vi "PH_ImageOperator.panel.vi"(0 "object ref":refnum<vi>, 5 "error in (no error)":errorcluster) -> (19 "error out":errorcluster)   [LabVIEW 2014, in "PH_ImageOperator.lvlib"]
doc: "The voltage measured by a device on high potential is represented by a frequency given out by a Beckhoff Klemme. This VI transforms it back into a voltage which wich is written to a memory tag. This value is indicated. In case of no connection (not mounted or bad tag value) or internal problems \"99999\" apears.\n\n\"Exit\" closes the GUI while \"Delete Instance\" additionally destroys the Instance.\n\n\n\nLicense Agreement for this software:\n\nCopyright (C)\nGesellschaft für Schwerionenforschung, GSI\nPlanckstr. 1\n64291 Darmstadt\nGermany\n\nContact: D.Beck@gsi.de \n\nThis program is free software; you can redistribute it and/or modify it under the terms of the GNU General Public License as published by the Free Software Foundation; either version 2 of the license, or (at your option) any later version.\n\nThis program is distributed in the hope that it will be useful, but WITHOUT ANYW ARRANTY; without even the implied warranty of MERCHANTABILITY or FITNESS FOR A PARTICULAR PURPOSE. See the GNU General License for more details (http://www.gnu.org).\n\nGesellschaft für Schwerionenforschung, GSI\nPlanckstr. 1, 64291 Darmstadt, Germany\nFor all questions and ideas contact: M.Richter@gsi.de, H.Brand@gsi.de or D.Beck@gsi.de.\nLast update: 18-DEC-2002"
uses:
  PH_ImageOperator.lvlib
  PH_ImageCalibrator/PH_ImageCalibrator.Calibration Data.ctl
  PH_Basics/PH_Img_BaseClass/PH_Img_BaseClass.Palette.ctl
  PH_Basics/PH_Img_BaseClass/PH_Img_BaseClass.GUI Refs.ctl
  CS_Core/CSObj/CSObj.lvlib
  CS_Core/CSSystem/CSSystemLib/CSSystemLib.lvlib
  PH_Basics/PH_Common/PH_Common.lvlib
  PH_Basics/PH_Img_BaseClass/PH_Img_BaseClass.lvlib
  PH_Basics/PH_Class/PH_Class.lvlib
  PH_Basics/PH_PSDBWriter/PH_PSDBWriter.lvlib
  PH_ImageCalibrator/PH_ImageCalibrator.lvlib
panel:
  out "PSDB Status":u32(colorbox)=6618880 caption="PSDB"
  in  "M":dbl
  in  "f 2":dbl caption="mm"
  out "Calibration status":u32(colorbox)=16860 caption="Calibration"
  out "Timeout":u32(colorbox)=16860
  in  "Tab Control":T1(tab)
  in  "Filter":bool
  in  "Damage Threshold":dbl=3.0 caption="J/cm²"
  in  "FF: Threshold":dbl=0.13 caption="Threshold"
  out "max. allowed Energy":dbl caption="J"
  out "Fillfactor":dbl
  out "Fill Factor calculated":u32(colorbox)=16860 caption="Fill Factor"
  in  "calc Fill Factor":bool caption="Fill Factor"
  out "Min 1 %":dbl caption="Pix"
  out "Maj 1 %":dbl caption="Pix"
  in  "Traces: No Offset":bool caption="No Offset"
  out "Traces calculated":u32(colorbox)=16860 caption="Trace"
  in  "Traces: Fit Gauss":bool caption="Fit Gauss"
  out "Min Fit Order":i32
  out "Maj Fit Order":i32
  out "Min FWHM":dbl caption="Pix"
  out "Maj FWHM":dbl caption="Pix"
  in  "Traces":bool
  in  "Timeout Set":i32 caption="ms"
  in  "Global On":bool caption="On"
  out "BI subtracted":u32(colorbox)=16860
  out "D":dbl caption="mm"
  out "q":dbl caption="mrad"
  in  "Center":bool
  in  "exp - Y":i32 caption="Pix"
  in  "Tolerance":dbl caption="mrad"
  in  "exp - X":i32 caption="Pix"
  out "Position calculated":u32(colorbox)=16860 caption="Position"
  in  "Type":bool
  in  "Position":bool
  out "Dummy Type":bool caption="NF       FF"
  in  "BA: Method":bool caption="Method"
  in  "BA: Factor for ROI":i32=3 caption="Factor"
  in  "BA: Steps":i32=3 caption="Steps"
  out "CoG - Y":dbl caption="Pix"
  out "CoG - X":dbl caption="Pix"
  out "e":dbl caption="PixSum"
  out "f":dbl caption="°"
  out "Min Diam":dbl caption="Pix"
  out "Maj Diam":dbl caption="Pix"
  out "Beam analysed":u32(colorbox)=16860 caption="Beam Analysis"
  in  "calc Beam Analysis":bool caption="Analysis"
  out "Dummy Method":bool caption="OA     ROI"
  out "Energy":dbl caption="PiS" format="%#_8g"
  out "Energy calculated":u32(colorbox)=16860 caption="Energy"
  in  "Tolerance":dbl caption="%"
  in  "expected":dbl caption="mJ"
  in  "calc Energy":bool caption="Energy"
  out "Minor Trace":cluster{"Index":sgl[], dbl[]}[](graph)
  out "Major Trace":cluster{"Index":sgl[], dbl[]}[](graph)
  in  "Palette":T2 items=["Grey", "Binary", "Gradient", "Rainbow", "Temperature"]
  out "GUI Image":T3(plugin-control)
  out "GUI FF Image":T3(plugin-control)
  in  "read calibration data":bool
  out "Calibration data":T4
  in  "Exit":bool
  in  "Delete":bool
  # "PCS"
  # "3.40"
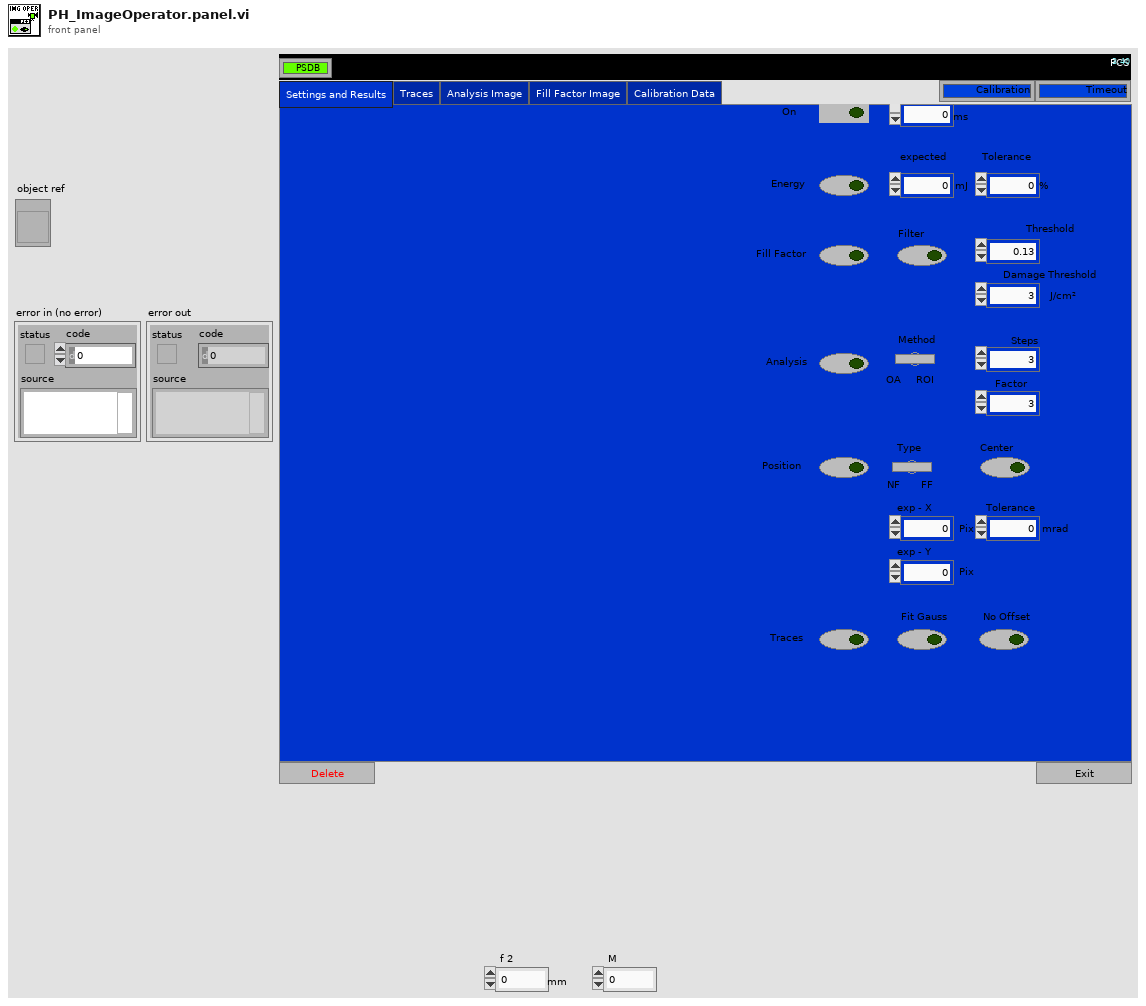
[diagram p1: front panel]
types:
  T1 = enum32{"Settings and Results", "Traces", "Analysis Image", "Fill Factor Image", "Calibration Data"}
  T2 = typedef "PH_Img_BaseClass.lvlib/PH_Img_BaseClass.Palette.ctl" = i32
  T3 = typedef "IMAQ Image.ctl" = refnum<image>
  T4 = typedef "PH_ImageCalibrator.lvlib/PH_ImageCalibrator.Calibration Data.ctl" = cluster{"Date":string, "Time":string, "Cam Settings":cluster{"Cam ID":string, "Gain":dbl, "Brightness":dbl, "Shutter":dbl, "Cam Error":bool, "Mode":i32}, "Background Image":cluster{"Image":dbl[][], "Image Error":bool}, "Linear Calibration":cluster{"Calibration Factor":dbl, "not mm or mrad":bool}, "Energy Calibration":cluster{"Calibration Factor":dbl, "no mJ":bool}}
  T5 = typedef "PH_Img_BaseClass.lvlib/PH_Img_BaseClass.GUI Refs.ctl" = cluster{"Timeout":refnum<vi>, "Image":refnum<vi>, "Palette":refnum<vi>, "Timeout Set":refnum<vi>}
  T6 = typedef "PH_ImageOperator.lvlib/PH_ImageOperator.i attribute.ctl" = cluster{"GUI Refs":cluster{"Delete":refnum<vi>, "Calibration status":refnum<vi>, "BI subtracted":refnum<vi>, "calc Energy":refnum<vi>, "Energy: expected value":refnum<vi>, "Energy: Tolerance":refnum<vi>, "Energy calculated":refnum<vi>, "Energy":refnum<vi>, "calc Beam Anal":refnum<vi>, "Maj Diam 1/esquare":refnum<vi>, "Min Diam 1/esquare":refnum<vi>, "Azi Angle":refnum<vi>, "Min/Maj Diam esquare":refnum<vi>, "Beam analysed":refnum<vi>, "CoG - x":refnum<vi>, "CoG - y":refnum<vi>, "BA: Method":refnum<vi>, "BA: Steps":refnum<vi>, "BA: Factor":refnum<vi>, "calc Traces":refnum<vi>, "Traces: Fit Gauss":refnum<vi>, "Traces calculated":refnum<vi>, "Maj FWHM":refnum<vi>, "Min FWHM":refnum<vi>, "Major Trace":refnum<vi>, "Minor Trace":refnum<vi>, "Maj Fit Order":refnum<vi>, "Min Fit Order":refnum<vi>, "Position calculated":refnum<vi>, "Position":refnum<vi>, "Type":refnum<vi>, "Center":refnum<vi>, "exp - X":refnum<vi>, "exp - Y":refnum<vi>, "Tolerance":refnum<vi>, "f":refnum<vi>, "M":refnum<vi>, "D":refnum<vi>, "q":refnum<vi>, "Dummy Method":refnum<vi>, "Dummy Type":refnum<vi>, "Global On":refnum<vi>, "Traces: No offset":refnum<vi>, "Maj 99%":refnum<vi>, "Min 99%":refnum<vi>, "GUI FF Image":refnum<vi>, "calc Fill Factor":refnum<vi>, "FF calculated":refnum<vi>, "Fill Factor: Filter?":refnum<vi>, "FF: Damage Threshold":refnum<vi>, "FF: Threshold":refnum<vi>, "FF: max allow. Energy":refnum<vi>, "FF: Fillfactor":refnum<vi>, "Calibration data":refnum<vi>}, "List of GUIs":string[], "Calibration":cluster{"Status":T7, "Calibration data":T4, "Calibration Data File":path}, "Final Image":cluster{"BI Subtraction Failure":bool}, "Energy":cluster{"on":bool, "expected value [mJ]":dbl, "Tolerance [%]":dbl, "State":T7, "Energy [mJ]":dbl, "Unit":string, "calculated @":timestamp}, "Beam Analysis":cluster{"on":bool, "Data":T8, "Method":bool, "Steps":i32, "Factor":i32, "ROI":cluster{"Left":i32, "Top":i32, "Right":i32, "Bottom":i32}, "analysed @":timestamp}, "Trace Analysis":cluster{"on":bool, "Fit on":bool, "Maj FWHM":dbl, "Min FWHM":dbl, "Maj Fit Order":i32, "Min Fit Order":i32, "No Offset":bool, "Maj 99%":dbl, "Min 99%":dbl, "Traces":cluster{"XScaleName":string, "Y Scale Minimum":sgl, "Y Scale Maximum":sgl, "X Scale Minimum":sgl, "X Scale Maximum":sgl, "Traces":cluster{"Index":sgl[], "Trace":dbl[]}[]}[], "analysed @":timestamp}, "Position Analysis":cluster{"on":bool, "exp - X":i32, "exp - Y":i32, "focal length [mm]":dbl, "Magnification":dbl, "Delta":dbl, "Theta":dbl, "Tolerance":dbl, "Type":bool, "analysed @":timestamp}, "Fill Factor":cluster{"on":bool, "Filter on?":bool, "Threshold":dbl, "Damage Threshold [J/cm²]":dbl, "Fillfactor":dbl, "Max. allowed Energy [J]":dbl, "calculated @":timestamp}, "Statistician Service ID":i32, "Images":cluster{"Background":T3, "OP":T3, "GUI":T3, "BA: ROI":T3, "Trace: Turn":T3, "FF: Main":T3, "FF: Help":T3, "PSDB: BG":T3, "PSDB: OP":T3, "PSDB: FF":T3}}
  T7 = typedef "PH_StatusHandler.lvlib/PH_StatusHandler.Status.ctl" = i16
  T8 = typedef "PH_ImageOperator.lvlib/PH_ImageOperator.Beam Analysis Data.ctl" = cluster{"CoG-x":sgl, "CoG-y":sgl, "Maj Dim":dbl, "Min Dim":dbl, "Ellipticity":dbl, "Azimuth Angle [rad]":dbl, "Azi Angle rel to Maj?":bool}
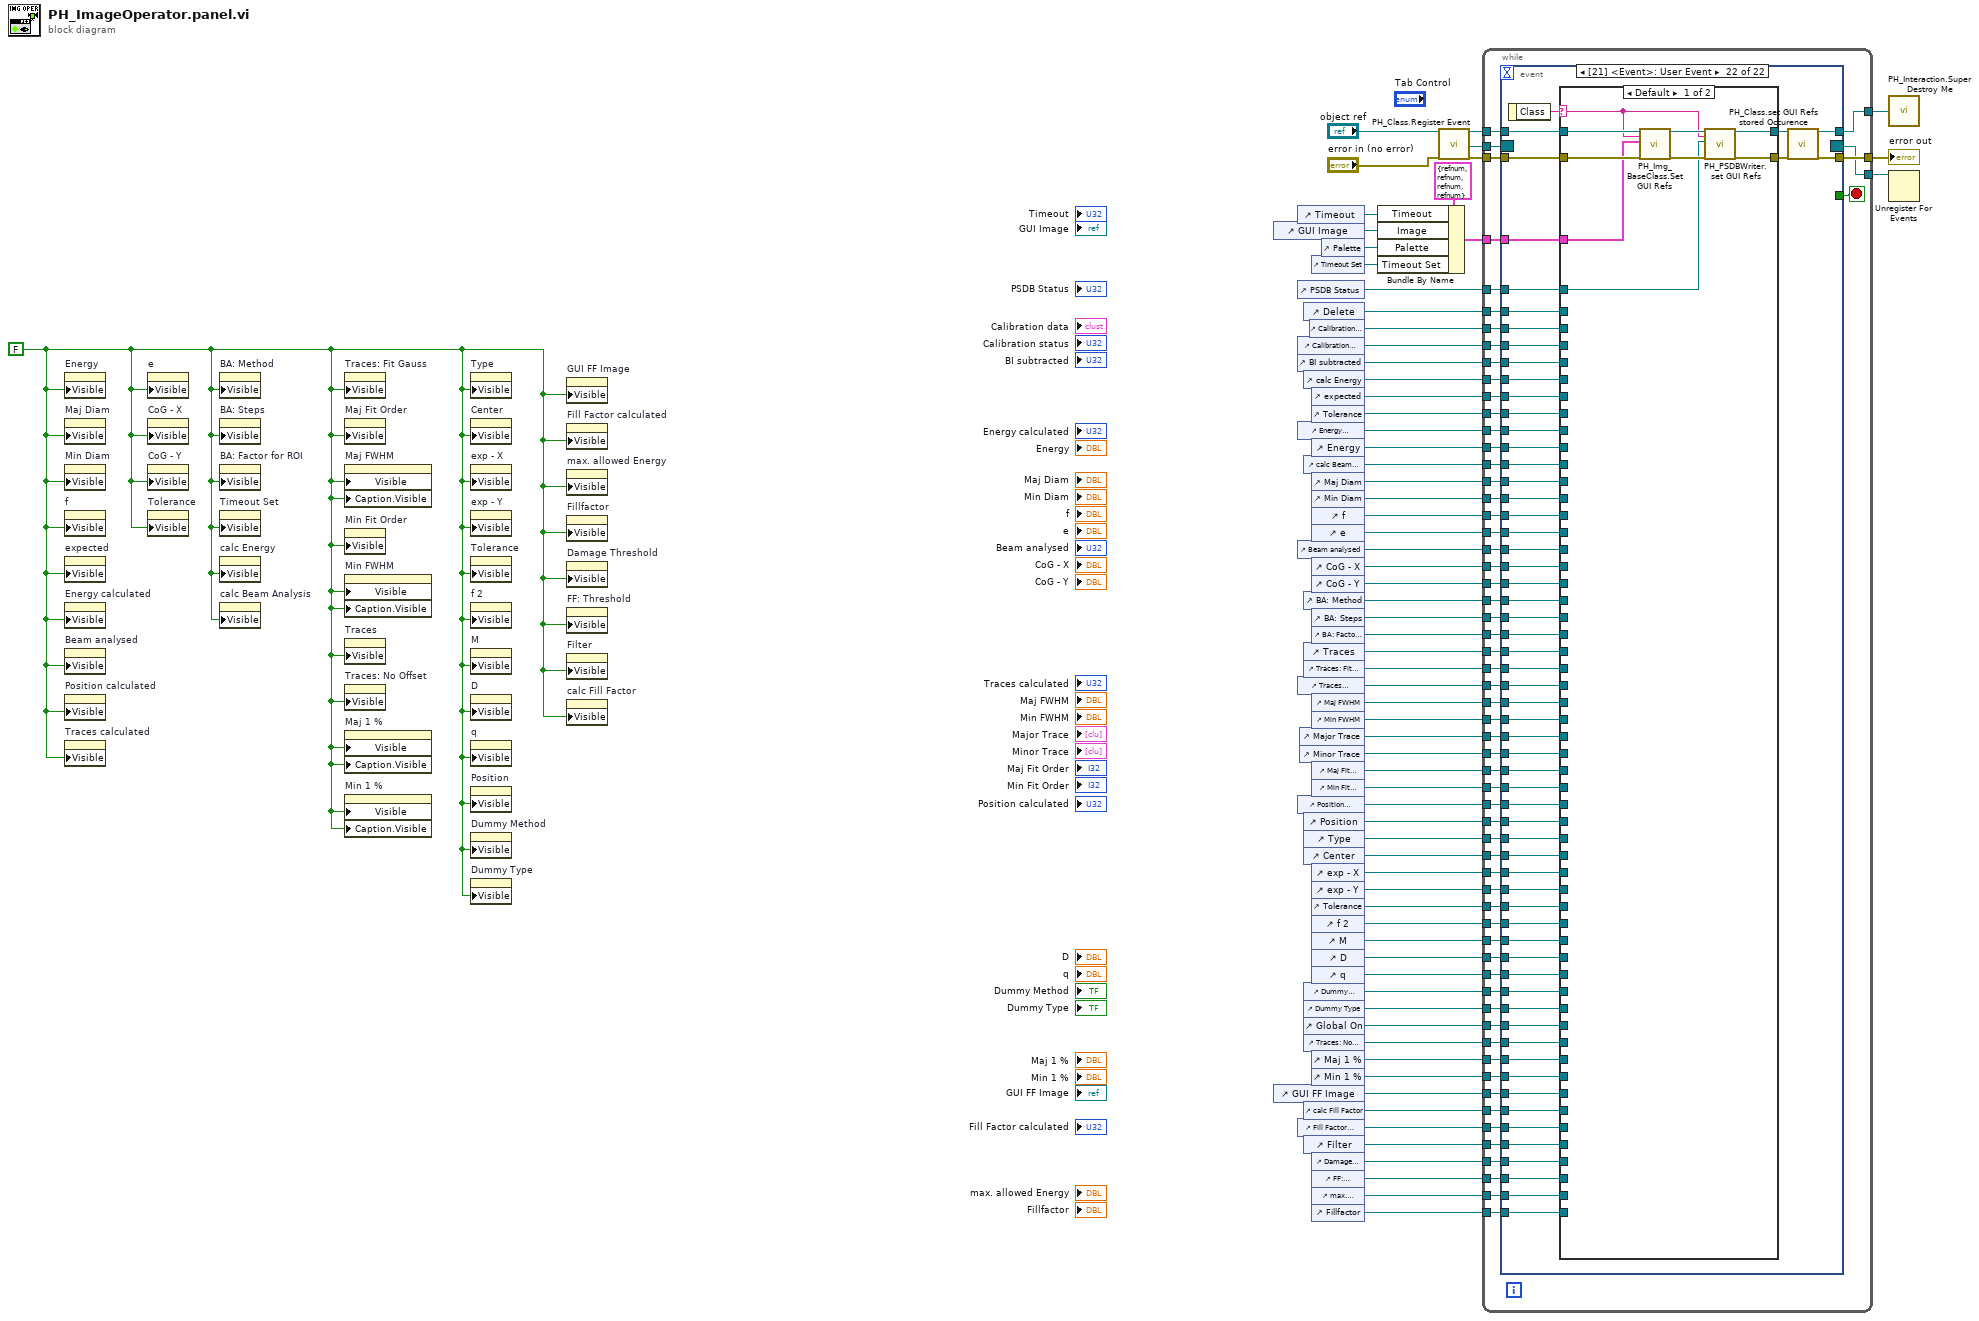
[diagram p0: block diagram]
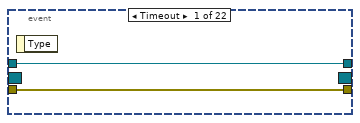
[diagram p2: hidden frame]
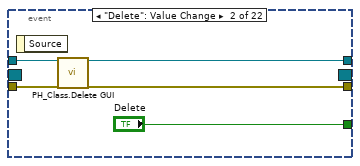
[diagram p3: hidden frame]
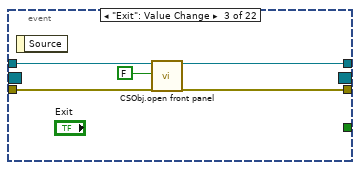
[diagram p4: hidden frame]
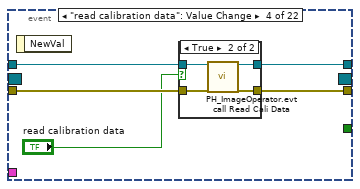
[diagram p5: hidden frame]
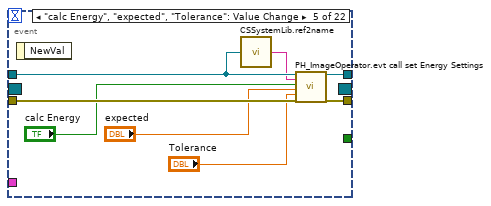
[diagram p7: hidden frame]
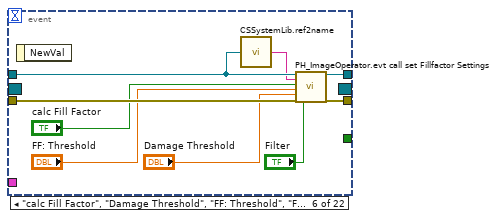
[diagram p8: hidden frame]
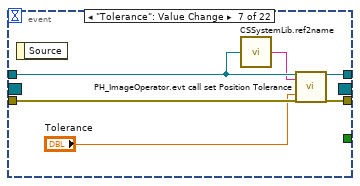
[diagram p9: hidden frame]
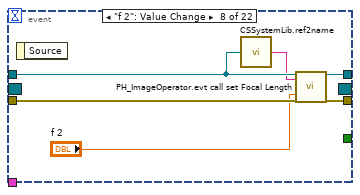
[diagram p10: hidden frame]
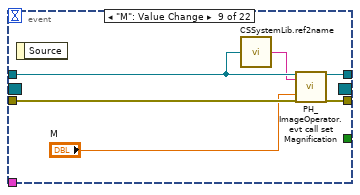
[diagram p11: hidden frame]
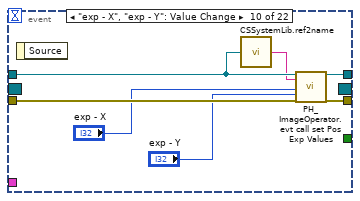
[diagram p12: hidden frame]
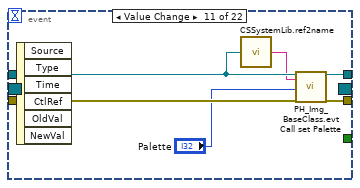
[diagram p13: hidden frame]
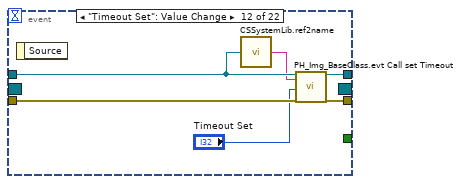
[diagram p14: hidden frame]
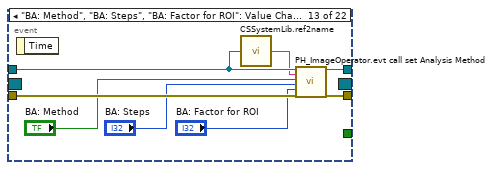
[diagram p15: hidden frame]
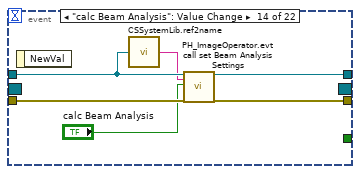
[diagram p16: hidden frame]
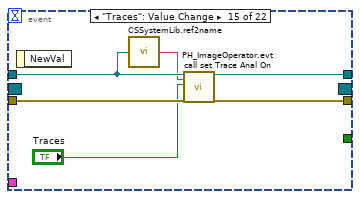
[diagram p17: hidden frame]
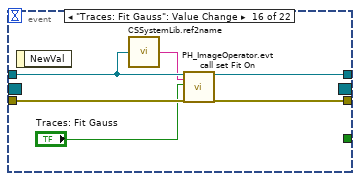
[diagram p18: hidden frame]
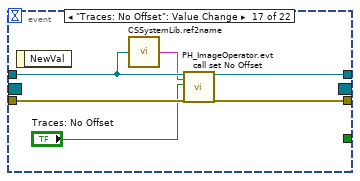
[diagram p19: hidden frame]
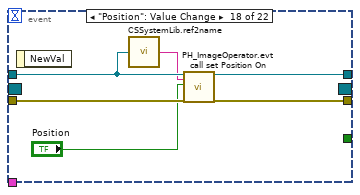
[diagram p20: hidden frame]
diagram:
  w68 = FALSE
  n1 = property on="Energy" class="DigNum (strict)"("Visible"=w68) -> ()  [unwired: 2 in, 2 out]
  n2 = property on="Maj Diam" class="DigNum (strict)"("Visible"=w68) -> ()  [unwired: 2 in, 2 out]
  n3 = property on="Min Diam" class="DigNum (strict)"("Visible"=w68) -> ()  [unwired: 2 in, 2 out]
  n4 = property on="f" class="DigNum (strict)"("Visible"=w68) -> ()  [unwired: 2 in, 2 out]
  n5 = property on="expected" class="DigNum (strict)"("Visible"=w68) -> ()  [unwired: 2 in, 2 out]
  n6 = property on="Energy calculated" class="ColBox"("Visible"=w68) -> ()  [unwired: 2 in, 2 out]
  n7 = property on="Beam analysed" class="ColBox"("Visible"=w68) -> ()  [unwired: 2 in, 2 out]
  n8 = property on="Position calculated" class="ColBox"("Visible"=w68) -> ()  [unwired: 2 in, 2 out]
  n9 = property on="Traces calculated" class="ColBox"("Visible"=w68) -> ()  [unwired: 2 in, 2 out]
  n10 = property on="e" class="DigNum (strict)"("Visible"=w68) -> ()  [unwired: 2 in, 2 out]
  n11 = property on="CoG - X" class="DigNum (strict)"("Visible"=w68) -> ()  [unwired: 2 in, 2 out]
  n12 = property on="CoG - Y" class="DigNum (strict)"("Visible"=w68) -> ()  [unwired: 2 in, 2 out]
  n13 = property on="Tolerance" class="DigNum (strict)"("Visible"=w68) -> ()  [unwired: 2 in, 2 out]
  n14 = property on="BA: Method" class="Bool (strict)"("Visible"=w68) -> ()  [unwired: 2 in, 2 out]
  n15 = property on="BA: Steps" class="DigNum (strict)"("Visible"=w68) -> ()  [unwired: 2 in, 2 out]
  n16 = property on="BA: Factor for ROI" class="DigNum (strict)"("Visible"=w68) -> ()  [unwired: 2 in, 2 out]
  n17 = property on="Timeout Set" class="DigNum (strict)"("Visible"=w68) -> ()  [unwired: 2 in, 2 out]
  n18 = property on="calc Energy" class="Bool (strict)"("Visible"=w68) -> ()  [unwired: 2 in, 2 out]
  n19 = property on="calc Beam Analysis" class="Bool (strict)"("Visible"=w68) -> ()  [unwired: 2 in, 2 out]
  n20 = property on="Traces: Fit Gauss" class="Bool (strict)"("Visible"=w68) -> ()  [unwired: 2 in, 2 out]
  n21 = property on="Maj Fit Order" class="DigNum (strict)"("Visible"=w68) -> ()  [unwired: 2 in, 2 out]
  n22 = property on="Maj FWHM" class="DigNum (strict)"("Visible"=w68, "Caption.Visible"=w68) -> ()  [unwired: 2 in, 2 out]
  n23 = property on="Min Fit Order" class="DigNum (strict)"("Visible"=w68) -> ()  [unwired: 2 in, 2 out]
  n24 = property on="Min FWHM" class="DigNum (strict)"("Visible"=w68, "Caption.Visible"=w68) -> ()  [unwired: 2 in, 2 out]
  n25 = property on="Traces" class="Bool (strict)"("Visible"=w68) -> ()  [unwired: 2 in, 2 out]
  n26 = property on="Traces: No Offset" class="Bool (strict)"("Visible"=w68) -> ()  [unwired: 2 in, 2 out]
  n27 = property on="Maj 1 %" class="DigNum (strict)"("Visible"=w68, "Caption.Visible"=w68) -> ()  [unwired: 2 in, 2 out]
  n28 = property on="Min 1 %" class="DigNum (strict)"("Visible"=w68, "Caption.Visible"=w68) -> ()  [unwired: 2 in, 2 out]
  n29 = property on="Type" class="Bool (strict)"("Visible"=w68) -> ()  [unwired: 2 in, 2 out]
  n30 = property on="Center" class="Bool (strict)"("Visible"=w68) -> ()  [unwired: 2 in, 2 out]
  n31 = property on="exp - X" class="DigNum (strict)"("Visible"=w68) -> ()  [unwired: 2 in, 2 out]
  n32 = property on="exp - Y" class="DigNum (strict)"("Visible"=w68) -> ()  [unwired: 2 in, 2 out]
  n33 = property on="Tolerance" class="DigNum (strict)"("Visible"=w68) -> ()  [unwired: 2 in, 2 out]
  n34 = property on="f 2" class="DigNum (strict)"("Visible"=w68) -> ()  [unwired: 2 in, 2 out]
  n35 = property on="M" class="DigNum (strict)"("Visible"=w68) -> ()  [unwired: 2 in, 2 out]
  n36 = property on="D" class="DigNum (strict)"("Visible"=w68) -> ()  [unwired: 2 in, 2 out]
  n37 = property on="q" class="DigNum (strict)"("Visible"=w68) -> ()  [unwired: 2 in, 2 out]
  n38 = property on="Position" class="Bool (strict)"("Visible"=w68) -> ()  [unwired: 2 in, 2 out]
  n39 = property on="Dummy Method" class="Bool (strict)"("Visible"=w68) -> ()  [unwired: 2 in, 2 out]
  n40 = property on="Dummy Type" class="Bool (strict)"("Visible"=w68) -> ()  [unwired: 2 in, 2 out]
  n41 = property on="GUI FF Image" class="ImageControl"("Visible"=w68) -> ()  [unwired: 2 in, 2 out]
  n42 = property on="Fill Factor calculated" class="ColBox"("Visible"=w68) -> ()  [unwired: 2 in, 2 out]
  n43 = property on="max. allowed Energy" class="DigNum (strict)"("Visible"=w68) -> ()  [unwired: 2 in, 2 out]
  n44 = property on="Fillfactor" class="DigNum (strict)"("Visible"=w68) -> ()  [unwired: 2 in, 2 out]
  n45 = property on="Damage Threshold" class="DigNum (strict)"("Visible"=w68) -> ()  [unwired: 2 in, 2 out]
  n46 = property on="FF: Threshold" class="DigNum (strict)"("Visible"=w68) -> ()  [unwired: 2 in, 2 out]
  n47 = property on="Filter" class="Bool (strict)"("Visible"=w68) -> ()  [unwired: 2 in, 2 out]
  n48 = property on="calc Fill Factor" class="Bool (strict)"("Visible"=w68) -> ()  [unwired: 2 in, 2 out]
  n49 = control-ref of="GUI Image"() -> (w65:refnum<vi>)
  n50 = control-ref of="GUI FF Image"() -> (w8:refnum<vi>)
  n51 = control-ref of="Timeout"() -> (w66:refnum<vi>)
  n52 = control-ref of="PSDB Status"() -> (w57:refnum<vi>)
  n53 = control-ref of="Calibration status"() -> (w52:refnum<vi>)
  n54 = control-ref of="BI subtracted"() -> (w51:refnum<vi>)
  n55 = control-ref of="Energy calculated"() -> (w47:refnum<vi>)
  n56 = control-ref of="Beam analysed"() -> (w40:refnum<vi>)
  n57 = control-ref of="Traces calculated"() -> (w32:refnum<vi>)
  n58 = control-ref of="Position calculated"() -> (w25:refnum<vi>)
  n59 = control-ref of="Fill Factor calculated"() -> (w6:refnum<vi>)
  n60 = control-ref of="Major Trace"() -> (w29:refnum<vi>)
  n61 = control-ref of="Minor Trace"() -> (w28:refnum<vi>)
  n62 = control-ref of="Delete"() -> (w56:refnum<vi>)
  n63 = control-ref of="calc Energy"() -> (w50:refnum<vi>)
  n64 = control-ref of="calc Beam Analysis"() -> (w45:refnum<vi>)
  n65 = control-ref of="BA: Method"() -> (w37:refnum<vi>)
  n66 = control-ref of="Traces"() -> (w34:refnum<vi>)
  n67 = control-ref of="Traces: Fit Gauss"() -> (w33:refnum<vi>)
  n68 = control-ref of="Position"() -> (w24:refnum<vi>)
  n69 = control-ref of="Type"() -> (w23:refnum<vi>)
  n70 = control-ref of="Center"() -> (w22:refnum<vi>)
  n71 = control-ref of="Dummy Method"() -> (w14:refnum<vi>)
  n72 = control-ref of="Dummy Type"() -> (w13:refnum<vi>)
  n73 = control-ref of="Global On"() -> (w12:refnum<vi>)
  n74 = control-ref of="Traces: No Offset"() -> (w11:refnum<vi>)
  n75 = control-ref of="calc Fill Factor"() -> (w7:refnum<vi>)
  n76 = control-ref of="Filter"() -> (w5:refnum<vi>)
  n77 = control-ref of="Calibration data"() -> (w53:refnum<vi>)
  n78 = control-ref of="Timeout Set"() -> (w63:refnum<vi>)
  n79 = control-ref of="expected"() -> (w49:refnum<vi>)
  n80 = control-ref of="Tolerance"() -> (w48:refnum<vi>)
  n81 = control-ref of="Energy"() -> (w46:refnum<vi>)
  n82 = control-ref of="Maj Diam"() -> (w44:refnum<vi>)
  n83 = control-ref of="Min Diam"() -> (w43:refnum<vi>)
  n84 = control-ref of="f"() -> (w42:refnum<vi>)
  n85 = control-ref of="e"() -> (w41:refnum<vi>)
  n86 = control-ref of="CoG - X"() -> (w39:refnum<vi>)
  n87 = control-ref of="CoG - Y"() -> (w38:refnum<vi>)
  n88 = control-ref of="BA: Steps"() -> (w36:refnum<vi>)
  n89 = control-ref of="BA: Factor for ROI"() -> (w35:refnum<vi>)
  n90 = control-ref of="Maj FWHM"() -> (w31:refnum<vi>)
  n91 = control-ref of="Min FWHM"() -> (w30:refnum<vi>)
  n92 = control-ref of="Maj Fit Order"() -> (w27:refnum<vi>)
  n93 = control-ref of="Min Fit Order"() -> (w26:refnum<vi>)
  n94 = control-ref of="exp - X"() -> (w21:refnum<vi>)
  n95 = control-ref of="exp - Y"() -> (w20:refnum<vi>)
  n96 = control-ref of="Tolerance"() -> (w19:refnum<vi>)
  n97 = control-ref of="f 2"() -> (w18:refnum<vi>)
  n98 = control-ref of="M"() -> (w17:refnum<vi>)
  n99 = control-ref of="D"() -> (w16:refnum<vi>)
  n100 = control-ref of="q"() -> (w15:refnum<vi>)
  n101 = control-ref of="Maj 1 %"() -> (w10:refnum<vi>)
  n102 = control-ref of="Min 1 %"() -> (w9:refnum<vi>)
  n103 = control-ref of="Damage Threshold"() -> (w4:refnum<vi>)
  n104 = control-ref of="FF: Threshold"() -> (w3:refnum<vi>)
  n105 = control-ref of="max. allowed Energy"() -> (w2:refnum<vi>)
  n106 = control-ref of="Fillfactor"() -> (w1:refnum<vi>)
  n107 = control-ref of="Palette"() -> (w64:refnum<vi>)
  n108 = Bundle By Name(cluster=T5 {"Timeout"=refnum, "Image"=refnum, "Palette"=refnum, "Timeout Set"=refnum} ("GUI Refs"), "Timeout"=w66, "Image"=w65, "Palette"=w64, "Timeout Set"=w63) -> (w58:T5)
  n109 = call "PH_Class.Register Event.vi"("i ref in"="object ref", "error in (no error)"="error in (no error)") -> ("i ref out"=w60:refnum<vi>, "Event Registration Refnum"=w59:refnum<event-registration>, "error out"=w61:errorcluster)  [unwired: 15 in]
  n110 = while {
    tunnel: w60 -> [w130]
    tunnel: [w129] -> w70
    tunnel: w61 -> [w132]
    tunnel: [w131] -> w69
    tunnel: [w128] -> w62
    tunnel: w59 -> [w127]
    tunnel: w58 -> [w126]
    tunnel: w57 -> [w125]
    tunnel: w56 -> [w124]
    tunnel: w53 -> [w123]
    tunnel: w52 -> [w122]
    tunnel: w51 -> [w121]
    tunnel: w50 -> [w120]
    tunnel: w49 -> [w119]
    tunnel: w48 -> [w118]
    tunnel: w47 -> [w117]
    tunnel: w46 -> [w116]
    tunnel: w45 -> [w115]
    tunnel: w44 -> [w114]
    tunnel: w43 -> [w113]
    tunnel: w42 -> [w112]
    tunnel: w41 -> [w111]
    tunnel: w40 -> [w110]
    tunnel: w39 -> [w109]
    tunnel: w38 -> [w108]
    tunnel: w37 -> [w107]
    tunnel: w36 -> [w106]
    tunnel: w35 -> [w105]
    tunnel: w34 -> [w104]
    tunnel: w33 -> [w103]
    tunnel: w32 -> [w102]
    tunnel: w31 -> [w101]
    tunnel: w30 -> [w100]
    tunnel: w29 -> [w99]
    tunnel: w28 -> [w98]
    tunnel: w27 -> [w97]
    tunnel: w26 -> [w96]
    tunnel: w25 -> [w95]
    tunnel: w24 -> [w94]
    tunnel: w23 -> [w93]
    tunnel: w22 -> [w92]
    tunnel: w21 -> [w91]
    tunnel: w20 -> [w90]
    tunnel: w19 -> [w89]
    tunnel: w18 -> [w88]
    tunnel: w17 -> [w87]
    tunnel: w16 -> [w86]
    tunnel: w15 -> [w85]
    tunnel: w14 -> [w84]
    tunnel: w13 -> [w83]
    tunnel: w12 -> [w82]
    tunnel: w11 -> [w81]
    tunnel: w10 -> [w80]
    tunnel: w9 -> [w79]
    tunnel: w8 -> [w78]
    tunnel: w7 -> [w77]
    tunnel: w6 -> [w76]
    tunnel: w5 -> [w75]
    tunnel: w4 -> [w74]
    tunnel: w3 -> [w73]
    tunnel: w2 -> [w72]
    tunnel: w1 -> [w71]
    stop <- w133 stop-if-true
    n111 = event shown="[21] <Event>: User Event" {
      selector: w127 -> [_ _ _ _ _ _ _ _ _ _ _ _ _ _ _ _ _ _ _ _ _ _]
      dyn-events: [_ _ _ _ _ _ _ _ _ _ _ _ _ _ _ _ _ _ _ _ _ _] -> w128
      timeout: _ -> [_ _ _ _ _ _ _ _ _ _ _ _ _ _ _ _ _ _ _ _ _ _]
      tunnel: [_ "Delete" _ _ _ _ _ _ _ _ _ _ _ _ _ _ _ _ _ _ _ _] -> w133
      tunnel: w130 -> [w134 w138 w144 w150 w161 w170 w176 w182 w188 w195 w201 w207 w215 w221 w227 w233 w239 w245 w251 w257 w262 w328]
      tunnel: w132 -> [w135 w139 w143 w149 w164 w173 w179 w185 w191 w198 w204 w210 w218 w224 w230 w236 w242 w248 w254 w260 w265 w325]
      tunnel: [w135 w136 w142 w147 w162 w171 w177 w183 w189 w196 w202 w208 w216 w222 w228 w234 w240 w246 w252 w258 w263 w323] -> w131
      tunnel: [w134 w137 w141 w148 w163 w172 w178 w184 w190 w197 w203 w209 w217 w223 w229 w235 w241 w247 w253 w259 w264 w326] -> w129
      tunnel: w126 -> [_ _ _ _ _ _ _ _ _ _ _ _ _ _ _ _ _ _ _ _ _ w321]
      tunnel: w125 -> [_ _ _ _ _ _ _ _ _ _ _ _ _ _ _ _ _ _ _ _ _ w320]
      tunnel: w124 -> [_ _ _ _ _ _ _ _ _ _ _ _ _ _ _ _ _ _ _ _ _ w319]
      tunnel: w123 -> [_ _ _ _ _ _ _ _ _ _ _ _ _ _ _ _ _ _ _ _ _ w318]
      tunnel: w122 -> [_ _ _ _ _ _ _ _ _ _ _ _ _ _ _ _ _ _ _ _ _ w317]
      tunnel: w121 -> [_ _ _ _ _ _ _ _ _ _ _ _ _ _ _ _ _ _ _ _ _ w316]
      tunnel: w120 -> [_ _ _ _ _ _ _ _ _ _ _ _ _ _ _ _ _ _ _ _ _ w315]
      tunnel: w119 -> [_ _ _ _ _ _ _ _ _ _ _ _ _ _ _ _ _ _ _ _ _ w314]
      tunnel: w118 -> [_ _ _ _ _ _ _ _ _ _ _ _ _ _ _ _ _ _ _ _ _ w313]
      tunnel: w117 -> [_ _ _ _ _ _ _ _ _ _ _ _ _ _ _ _ _ _ _ _ _ w312]
      tunnel: w116 -> [_ _ _ _ _ _ _ _ _ _ _ _ _ _ _ _ _ _ _ _ _ w311]
      tunnel: w115 -> [_ _ _ _ _ _ _ _ _ _ _ _ _ _ _ _ _ _ _ _ _ w310]
      tunnel: w114 -> [_ _ _ _ _ _ _ _ _ _ _ _ _ _ _ _ _ _ _ _ _ w309]
      tunnel: w113 -> [_ _ _ _ _ _ _ _ _ _ _ _ _ _ _ _ _ _ _ _ _ w308]
      tunnel: w112 -> [_ _ _ _ _ _ _ _ _ _ _ _ _ _ _ _ _ _ _ _ _ w307]
      tunnel: w111 -> [_ _ _ _ _ _ _ _ _ _ _ _ _ _ _ _ _ _ _ _ _ w306]
      tunnel: w110 -> [_ _ _ _ _ _ _ _ _ _ _ _ _ _ _ _ _ _ _ _ _ w305]
      tunnel: w109 -> [_ _ _ _ _ _ _ _ _ _ _ _ _ _ _ _ _ _ _ _ _ w304]
      tunnel: w108 -> [_ _ _ _ _ _ _ _ _ _ _ _ _ _ _ _ _ _ _ _ _ w303]
      tunnel: w107 -> [_ _ _ _ _ _ _ _ _ _ _ _ _ _ _ _ _ _ _ _ _ w302]
      tunnel: w106 -> [_ _ _ _ _ _ _ _ _ _ _ _ _ _ _ _ _ _ _ _ _ w301]
      tunnel: w105 -> [_ _ _ _ _ _ _ _ _ _ _ _ _ _ _ _ _ _ _ _ _ w300]
      tunnel: w104 -> [_ _ _ _ _ _ _ _ _ _ _ _ _ _ _ _ _ _ _ _ _ w299]
      tunnel: w103 -> [_ _ _ _ _ _ _ _ _ _ _ _ _ _ _ _ _ _ _ _ _ w298]
      tunnel: w102 -> [_ _ _ _ _ _ _ _ _ _ _ _ _ _ _ _ _ _ _ _ _ w297]
      tunnel: w101 -> [_ _ _ _ _ _ _ _ _ _ _ _ _ _ _ _ _ _ _ _ _ w296]
      tunnel: w100 -> [_ _ _ _ _ _ _ _ _ _ _ _ _ _ _ _ _ _ _ _ _ w295]
      tunnel: w99 -> [_ _ _ _ _ _ _ _ _ _ _ _ _ _ _ _ _ _ _ _ _ w294]
      tunnel: w98 -> [_ _ _ _ _ _ _ _ _ _ _ _ _ _ _ _ _ _ _ _ _ w293]
      tunnel: w97 -> [_ _ _ _ _ _ _ _ _ _ _ _ _ _ _ _ _ _ _ _ _ w292]
      tunnel: w96 -> [_ _ _ _ _ _ _ _ _ _ _ _ _ _ _ _ _ _ _ _ _ w291]
      tunnel: w95 -> [_ _ _ _ _ _ _ _ _ _ _ _ _ _ _ _ _ _ _ _ _ w290]
      tunnel: w94 -> [_ _ _ _ _ _ _ _ _ _ _ _ _ _ _ _ _ _ _ _ _ w289]
      tunnel: w93 -> [_ _ _ _ _ _ _ _ _ _ _ _ _ _ _ _ _ _ _ _ _ w288]
      tunnel: w92 -> [_ _ _ _ _ _ _ _ _ _ _ _ _ _ _ _ _ _ _ _ _ w287]
      tunnel: w91 -> [_ _ _ _ _ _ _ _ _ _ _ _ _ _ _ _ _ _ _ _ _ w286]
      tunnel: w90 -> [_ _ _ _ _ _ _ _ _ _ _ _ _ _ _ _ _ _ _ _ _ w285]
      tunnel: w89 -> [_ _ _ _ _ _ _ _ _ _ _ _ _ _ _ _ _ _ _ _ _ w284]
      tunnel: w88 -> [_ _ _ _ _ _ _ _ _ _ _ _ _ _ _ _ _ _ _ _ _ w283]
      tunnel: w87 -> [_ _ _ _ _ _ _ _ _ _ _ _ _ _ _ _ _ _ _ _ _ w282]
      tunnel: w86 -> [_ _ _ _ _ _ _ _ _ _ _ _ _ _ _ _ _ _ _ _ _ w281]
      tunnel: w85 -> [_ _ _ _ _ _ _ _ _ _ _ _ _ _ _ _ _ _ _ _ _ w280]
      tunnel: w84 -> [_ _ _ _ _ _ _ _ _ _ _ _ _ _ _ _ _ _ _ _ _ w279]
      tunnel: w83 -> [_ _ _ _ _ _ _ _ _ _ _ _ _ _ _ _ _ _ _ _ _ w278]
      tunnel: w82 -> [_ _ _ _ _ _ _ _ _ _ _ _ _ _ _ _ _ _ _ _ _ w277]
      tunnel: w81 -> [_ _ _ _ _ _ _ _ _ _ _ _ _ _ _ _ _ _ _ _ _ w276]
      tunnel: w80 -> [_ _ _ _ _ _ _ _ _ _ _ _ _ _ _ _ _ _ _ _ _ w275]
      tunnel: w79 -> [_ _ _ _ _ _ _ _ _ _ _ _ _ _ _ _ _ _ _ _ _ w274]
      tunnel: w78 -> [_ _ _ _ _ _ _ _ _ _ _ _ _ _ _ _ _ _ _ _ _ w273]
      tunnel: w77 -> [_ _ _ _ _ _ _ _ _ _ _ _ _ _ _ _ _ _ _ _ _ w272]
      tunnel: w76 -> [_ _ _ _ _ _ _ _ _ _ _ _ _ _ _ _ _ _ _ _ _ w271]
      tunnel: w75 -> [_ _ _ _ _ _ _ _ _ _ _ _ _ _ _ _ _ _ _ _ _ w270]
      tunnel: w74 -> [_ _ _ _ _ _ _ _ _ _ _ _ _ _ _ _ _ _ _ _ _ w269]
      tunnel: w73 -> [_ _ _ _ _ _ _ _ _ _ _ _ _ _ _ _ _ _ _ _ _ w268]
      tunnel: w72 -> [_ _ _ _ _ _ _ _ _ _ _ _ _ _ _ _ _ _ _ _ _ w267]
      tunnel: w71 -> [_ _ _ _ _ _ _ _ _ _ _ _ _ _ _ _ _ _ _ _ _ w266]
      event Timeout {
        n112 = event-data() -> ()  [unwired: 1 in, 1 out]
      }
      event "Delete": Value Change {
        n113 = event-data() -> ()  [unwired: 1 in, 1 out]
        n114 = call "PH_Class.Delete GUI.vi"("VI in"=w138, "error in (no error)"=w139) -> ("VI out"=w137:refnum<vi>, "error out"=w136:errorcluster)  [unwired: 16 in]
      }
      event "Exit": Value Change {
        n115 = event-data() -> ()  [unwired: 1 in, 1 out]
        n116 = call "CSObj.open front panel.vi"("i ref in"=w144, "frontPanelOpen"=FALSE ("front panel open"), "error in (no error)"=w143) -> ("i ref out"=w141:refnum<vi>, "error out"=w142:errorcluster)  [unwired: 15 in]
      }
      event "read calibration data": Value Change {
        n117 = event-data() -> ()  [unwired: 1 in, 1 out]
        n118 = case shown="True" "read calibration data" {
          tunnel: w150 -> [w152 w156]
          tunnel: w149 -> [w151 w155]
          tunnel: [w152 w154] -> w148
          tunnel: [w151 w153] -> w147
          frame False {
          }
          frame True {
            n119 = call "PH_ImageOperator.evt call Read Cali Data.vi"("i ref in"=w156, "error in"=w155) -> ("i ref out"=w154:refnum<vi>, "error out"=w153:errorcluster)  [unwired: 16 in]
          }
        }
      }
      event "calc Energy", "expected", "Tolerance": Value Change {
        n120 = event-data() -> ()  [unwired: 1 in, 1 out]
        n121 = call "CSSystemLib.ref2name.vi"("obj refnum"=w161) -> ("name"=w160:string)
        n122 = call "PH_ImageOperator.evt call set Energy Settings.vi"("i ref in"=w161, "Instance"=w160, "Calculate"="calc Energy", "expected value [mJ]"="expected", "Tolerance [%]"="Tolerance", "error in (no error)"=w164) -> ("i ref out"=w163:refnum<vi>, "error out"=w162:errorcluster)  [unwired: 12 in]
      }
      event "calc Fill Factor", "Damage Threshold", "FF: Threshold", "Filter": Value Change {
        n123 = event-data() -> ()  [unwired: 1 in, 1 out]
        n124 = call "CSSystemLib.ref2name.vi"("obj refnum"=w170) -> ("name"=w169:string)
        n125 = call "PH_ImageOperator.evt call set Fillfactor Settings.vi"("i ref in"=w170, "Instance"=w169, "Calculate"="calc Fill Factor", "Threshold"="FF: Threshold", "Damage Threshold [J/cm²]"="Damage Threshold", "error in (no error)"=w173, "Filter?"="Filter") -> ("i ref out"=w172:refnum<vi>, "error out"=w171:errorcluster)  [unwired: 11 in]
      }
      event "Tolerance": Value Change {
        n126 = event-data() -> ()  [unwired: 1 in, 1 out]
        n127 = call "CSSystemLib.ref2name.vi"("obj refnum"=w176) -> ("name"=w175:string)
        n128 = call "PH_ImageOperator.evt call set Position Tolerance.vi"("i ref in"=w176, "Instance"=w175, "Position Tolerance"="Tolerance", "error in (no error)"=w179) -> ("i ref out"=w178:refnum<vi>, "error out"=w177:errorcluster)  [unwired: 14 in]
      }
      event "f 2": Value Change {
        n129 = event-data() -> ()  [unwired: 1 in, 1 out]
        n130 = call "CSSystemLib.ref2name.vi"("obj refnum"=w182) -> ("name"=w181:string)
        n131 = call "PH_ImageOperator.evt call set Focal Length.vi"("i ref in"=w182, "Instance"=w181, "Focal Length"="f 2", "error in"=w185) -> ("i ref out"=w184:refnum<vi>, "error out"=w183:errorcluster)  [unwired: 14 in]
      }
      event "M": Value Change {
        n132 = event-data() -> ()  [unwired: 1 in, 1 out]
        n133 = call "CSSystemLib.ref2name.vi"("obj refnum"=w188) -> ("name"=w187:string)
        n134 = call "PH_ImageOperator.evt call set Magnification.vi"("i ref in"=w188, "Instance"=w187, "Magnification"="M", "error in"=w191) -> ("i ref out"=w190:refnum<vi>, "error out"=w189:errorcluster)  [unwired: 14 in]
      }
      event "exp - X", "exp - Y": Value Change {
        n135 = event-data() -> ()  [unwired: 1 in, 1 out]
        n136 = call "CSSystemLib.ref2name.vi"("obj refnum"=w195) -> ("name"=w194:string)
        n137 = call "PH_ImageOperator.evt call set Pos Exp Values.vi"("i ref in"=w195, "Instance"=w194, "expected value  x [Pix]"="exp - X", "expected value y [Pix]"="exp - Y", "error in (no error)"=w198) -> ("i ref out"=w197:refnum<vi>, "error out"=w196:errorcluster)  [unwired: 13 in]
      }
      event Value Change {
        n138 = event-data() -> ()  [unwired: 1 in, 6 out]
        n139 = call "CSSystemLib.ref2name.vi"("obj refnum"=w201) -> ("name"=w200:string)
        n140 = call "PH_Img_BaseClass.evt Call set Palette.vi"("i ref in"=w201, "Instance"=w200, "Palette"="Palette", "error in (no error)"=w204) -> ("i ref out"=w203:refnum<vi>, "error out"=w202:errorcluster)  [unwired: 14 in]
      }
      event "Timeout Set": Value Change {
        n141 = event-data() -> ()  [unwired: 1 in, 1 out]
        n142 = call "CSSystemLib.ref2name.vi"("obj refnum"=w207) -> ("name"=w206:string)
        n143 = call "PH_Img_BaseClass.evt Call set Timeout.vi"("i ref in"=w207, "Instance"=w206, "Timeout [ms]"="Timeout Set", "error in (no error)"=w210) -> ("i ref out"=w209:refnum<vi>, "error out"=w208:errorcluster)  [unwired: 14 in]
      }
      event "BA: Method", "BA: Steps", "BA: Factor for ROI": Value Change {
        n144 = event-data() -> ()  [unwired: 1 in, 1 out]
        n145 = call "CSSystemLib.ref2name.vi"("obj refnum"=w215) -> ("name"=w214:string)
        n146 = call "PH_ImageOperator.evt call set Analysis Method.vi"("i ref in"=w215, "Instance"=w214, "Method"="BA: Method", "Steps (3)"="BA: Steps", "Factor for ROI (3)"="BA: Factor for ROI", "error in (no error)"=w218) -> ("i ref out"=w217:refnum<vi>, "error out"=w216:errorcluster)  [unwired: 12 in]
      }
      event "calc Beam Analysis": Value Change {
        n147 = event-data() -> ()  [unwired: 1 in, 1 out]
        n148 = call "CSSystemLib.ref2name.vi"("obj refnum"=w221) -> ("name"=w220:string)
        n149 = call "PH_ImageOperator.evt call set Beam Analysis Settings.vi"("i ref in"=w221, "Instance"=w220, "Calculate"="calc Beam Analysis", "error in (no error)"=w224) -> ("i ref out"=w223:refnum<vi>, "error out"=w222:errorcluster)  [unwired: 14 in]
      }
      event "Traces": Value Change {
        n150 = event-data() -> ()  [unwired: 1 in, 1 out]
        n151 = call "CSSystemLib.ref2name.vi"("obj refnum"=w227) -> ("name"=w226:string)
        n152 = call "PH_ImageOperator.evt call set Trace Anal On.vi"("i ref in"=w227, "Instance"=w226, "Trace Anal on"="Traces", "error in (no error)"=w230) -> ("i ref out"=w229:refnum<vi>, "error out"=w228:errorcluster)  [unwired: 14 in]
      }
      event "Traces: Fit Gauss": Value Change {
        n153 = event-data() -> ()  [unwired: 1 in, 1 out]
        n154 = call "CSSystemLib.ref2name.vi"("obj refnum"=w233) -> ("name"=w232:string)
        n155 = call "PH_ImageOperator.evt call set Fit On.vi"("i ref in"=w233, "Instance"=w232, "Fit on"="Traces: Fit Gauss", "error in (no error)"=w236) -> ("i ref out"=w235:refnum<vi>, "error out"=w234:errorcluster)  [unwired: 14 in]
      }
      event "Traces: No Offset": Value Change {
        n156 = event-data() -> ()  [unwired: 1 in, 1 out]
        n157 = call "CSSystemLib.ref2name.vi"("obj refnum"=w239) -> ("name"=w238:string)
        n158 = call "PH_ImageOperator.evt call set No Offset.vi"("i ref in"=w239, "Instance"=w238, "No Offset"="Traces: No Offset", "error in (no error)"=w242) -> ("i ref out"=w241:refnum<vi>, "error out"=w240:errorcluster)  [unwired: 14 in]
      }
      event "Position": Value Change {
        n159 = event-data() -> ()  [unwired: 1 in, 1 out]
        n160 = call "CSSystemLib.ref2name.vi"("obj refnum"=w245) -> ("name"=w244:string)
        n161 = call "PH_ImageOperator.evt call set Position On.vi"("i ref in"=w245, "Instance"=w244, "Position On"="Position", "error in"=w248) -> ("i ref out"=w247:refnum<vi>, "error out"=w246:errorcluster)  [unwired: 14 in]
      }
      event "Type": Value Change {
        n162 = event-data() -> ()  [unwired: 1 in, 1 out]
        n163 = call "CSSystemLib.ref2name.vi"("obj refnum"=w251) -> ("name"=w250:string)
        n164 = call "PH_ImageOperator.evt call set Cam Type.vi"("i ref in"=w251, "Instance"=w250, "Cam Type"="Type", "error in (no error)"=w254) -> ("i ref out"=w253:refnum<vi>, "error out"=w252:errorcluster)  [unwired: 14 in]
      }
      event "Global On": Value Change {
        n165 = event-data() -> ()  [unwired: 1 in, 1 out]
        n166 = call "CSSystemLib.ref2name.vi"("obj refnum"=w257) -> ("name"=w256:string)
        n167 = call "PH_ImageOperator.evt call set Global On.vi"("i ref in"=w257, "Instance"=w256, "Global On"="Global On", "error in (no error)"=w260) -> ("i ref out"=w259:refnum<vi>, "error out"=w258:errorcluster)  [unwired: 14 in]
      }
      event "Center": Value Change {
        n168 = event-data() -> ()  [unwired: 1 in, 1 out]
        n169 = call "CSSystemLib.ref2name.vi"("obj refnum"=w262) -> ("name"=w261:string)
        n170 = call "PH_ImageOperator.evt call set Center.vi"("i ref in"=w262, "Instance"=w261, "error in (no error)"=w265) -> ("i ref out"=w264:refnum<vi>, "error out"=w263:errorcluster)  [unwired: 15 in]
      }
      event User Event {
        n171 = event-data() -> ("Class"=w322:string)  [unwired: 1 in]
        n172 = case shown="Default" w322 {
          selector: w322 -> [w330 _]
          tunnel: w328 -> [w337 w397]
          tunnel: [w333 w395] -> w327
          tunnel: w325 -> [w336 w396]
          tunnel: [w331 w394] -> w324
          tunnel: w321 -> [w335 _]
          tunnel: w320 -> [w329 _]
          tunnel: w319 -> [_ w391]
          tunnel: w318 -> [_ w390]
          tunnel: w317 -> [_ w389]
          tunnel: w316 -> [_ w388]
          tunnel: w315 -> [_ w387]
          tunnel: w314 -> [_ w386]
          tunnel: w313 -> [_ w385]
          tunnel: w312 -> [_ w384]
          tunnel: w311 -> [_ w383]
          tunnel: w310 -> [_ w382]
          tunnel: w309 -> [_ w381]
          tunnel: w308 -> [_ w380]
          tunnel: w307 -> [_ w379]
          tunnel: w306 -> [_ w378]
          tunnel: w305 -> [_ w377]
          tunnel: w304 -> [_ w376]
          tunnel: w303 -> [_ w375]
          tunnel: w302 -> [_ w374]
          tunnel: w301 -> [_ w373]
          tunnel: w300 -> [_ w372]
          tunnel: w299 -> [_ w371]
          tunnel: w298 -> [_ w370]
          tunnel: w297 -> [_ w369]
          tunnel: w296 -> [_ w368]
          tunnel: w295 -> [_ w367]
          tunnel: w294 -> [_ w366]
          tunnel: w293 -> [_ w365]
          tunnel: w292 -> [_ w364]
          tunnel: w291 -> [_ w363]
          tunnel: w290 -> [_ w362]
          tunnel: w289 -> [_ w361]
          tunnel: w288 -> [_ w360]
          tunnel: w287 -> [_ w359]
          tunnel: w286 -> [_ w358]
          tunnel: w285 -> [_ w357]
          tunnel: w284 -> [_ w356]
          tunnel: w283 -> [_ w355]
          tunnel: w282 -> [_ w354]
          tunnel: w281 -> [_ w353]
          tunnel: w280 -> [_ w352]
          tunnel: w279 -> [_ w351]
          tunnel: w278 -> [_ w350]
          tunnel: w277 -> [_ w349]
          tunnel: w276 -> [_ w348]
          tunnel: w275 -> [_ w347]
          tunnel: w274 -> [_ w346]
          tunnel: w273 -> [_ w345]
          tunnel: w272 -> [_ w344]
          tunnel: w271 -> [_ w343]
          tunnel: w270 -> [_ w342]
          tunnel: w269 -> [_ w341]
          tunnel: w268 -> [_ w340]
          tunnel: w267 -> [_ w339]
          tunnel: w266 -> [_ w338]
          frame Default {
            n173 = call "PH_Img_BaseClass.Set GUI Refs.vi"("i ref in"=w337, "Class"=w330, "GUI Refs"=w335, "error in (no error)"=w336) -> ("i ref out"=w334:refnum<vi>, "error out"=w332:errorcluster)  [unwired: 14 in]
            n174 = call "PH_PSDBWriter.set GUI Refs.vi"("i ref in"=w334, "Class"=w330, "Ref PSDB Status"=w329, "error in"=w332) -> ("i ref out"=w333:refnum<vi>, "error out"=w331:errorcluster)  [unwired: 14 in]
          }
          frame "PH_ImageOperator" {
            n175 = call "PH_ImageOperator.get data to modify.vi"("i ref in"=w397, "ms timeout (10000)"=-1, "error in (no error)"=w396) -> ("i ref out"=w398:refnum<vi>, "i attribute"=w393:T6, "error out"=w399:errorcluster)  [unwired: 13 in, 1 out]
            n176 = Bundle By Name(cluster=w393, "GUI Refs.Delete"=w391, "GUI Refs.Calibration data"=w390, "GUI Refs.Calibration status"=w389, "GUI Refs.BI subtracted"=w388, "GUI Refs.calc Energy"=w387, "GUI Refs.Energy: expected value"=w386, "GUI Refs.Energy: Tolerance"=w385, "GUI Refs.Energy calculated"=w384, "GUI Refs.Energy"=w383, "GUI Refs.calc Beam Anal"=w382, "GUI Refs.Maj Diam 1/esquare"=w381, "GUI Refs.Min Diam 1/esquare"=w380, "GUI Refs.Azi Angle"=w379, "GUI Refs.Min/Maj Diam esquare"=w378, "GUI Refs.Beam analysed"=w377, "GUI Refs.CoG - x"=w376, "GUI Refs.CoG - y"=w375, "GUI Refs.BA: Method"=w374, "GUI Refs.BA: Steps"=w373, "GUI Refs.BA: Factor"=w372, "GUI Refs.calc Traces"=w371, "GUI Refs.Traces: Fit Gauss"=w370, "GUI Refs.Traces calculated"=w369, "GUI Refs.Maj FWHM"=w368, "GUI Refs.Min FWHM"=w367, "GUI Refs.Major Trace"=w366, "GUI Refs.Minor Trace"=w365, "GUI Refs.Maj Fit Order"=w364, "GUI Refs.Min Fit Order"=w363, "GUI Refs.Position calculated"=w362, "GUI Refs.Position"=w361, "GUI Refs.Type"=w360, "GUI Refs.Center"=w359, "GUI Refs.exp - X"=w358, "GUI Refs.exp - Y"=w357, "GUI Refs.Tolerance"=w356, "GUI Refs.f"=w355, "GUI Refs.M"=w354, "GUI Refs.D"=w353, "GUI Refs.q"=w352, "GUI Refs.Dummy Method"=w351, "GUI Refs.Dummy Type"=w350, "GUI Refs.Global On"=w349, "GUI Refs.Traces: No offset"=w348, "GUI Refs.Maj 99%"=w347, "GUI Refs.Min 99%"=w346, "GUI Refs.GUI FF Image"=w345, "GUI Refs.calc Fill Factor"=w344, "GUI Refs.FF calculated"=w343, "GUI Refs.Fill Factor: Filter?"=w342, "GUI Refs.FF: Damage Threshold"=w341, "GUI Refs.FF: Threshold"=w340, "GUI Refs.FF: max allow. Energy"=w339, "GUI Refs.FF: Fillfactor"=w338) -> (w392:T6)
            n177 = call "PH_ImageOperator.set modified data.vi"("i ref in"=w398, "i attribute"=w392, "error in (no error)"=w399) -> ("i ref out"=w395:refnum<vi>, "error out"=w394:errorcluster)  [unwired: 15 in]
          }
        }
        n178 = call "PH_Class.set GUI Refs stored Occurence.vi"("i ref in"=w327, "error in (no error)"=w324) -> ("i ref out"=w326:refnum<vi>, "error out"=w323:errorcluster)  [unwired: 16 in]
      }
    }
  }
  "error out" <- w69
  n179 = call "PH_Interaction.Super Destroy Me.vi"("i ref out"=w70) -> ()
  n180 = Unregister For Events(event registration refnum=w62) -> ()  [unwired: 1 in, 1 out]
